vi "Initialize.vi"   [LabVIEW 2023, in "Longer Pump dLSP501 Series.lvlib"]
uses:
  <instrlib>/Longer Pump dLSP501 Modbus RTU Series/Longer Pump dLSP501 Series.lvlib
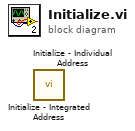
[diagram p0: block diagram]
diagram:
  n1 = call <instrlib>:"Initialize - Integrated Address.vi"() -> ()  [unwired: 8 in, 3 out]
  n2 = call <instrlib>:"Initialize - Individual Address.vi"() -> ()  [unwired: 8 in, 3 out]
